vi "controlArticular.vi"(4 "theta2Articular":dbl, 5 "theta1Articular":dbl, 6 "theta2":dbl, 7 "theta1":dbl, 9 "tiempoFinal":dbl, 10 "controlArticular":bool, 11 "tiempoArticular":dbl) -> (1 "tiempoFinal":dbl, 2 "theta2":dbl, 3 "theta1":dbl)   [LabVIEW 2019]
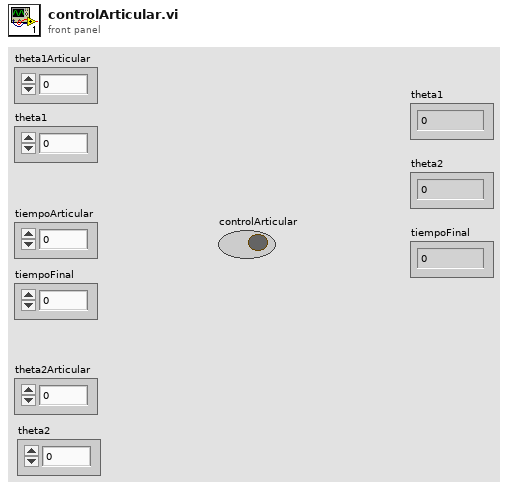
[diagram p1: front panel]
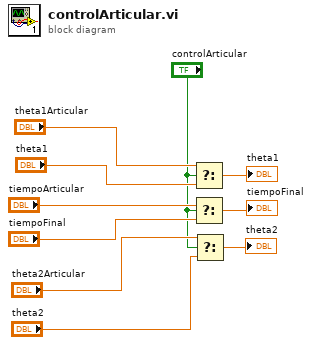
[diagram p0: block diagram]
diagram:
  n1 = Select(t="theta1Articular", s="controlArticular", f="theta1") -> (s? t:f=→"theta1":dbl)
  n2 = Select(t="tiempoArticular", s="controlArticular", f="tiempoFinal") -> (s? t:f=→"tiempoFinal":dbl)
  n3 = Select(t="theta2Articular", s="controlArticular", f="theta2") -> (s? t:f=→"theta2":dbl)
